vi "Shut_down_EnFlo_Tunnel.vi"(3 "Mode":T5=enum."Run VI", 5 "Traverse line In":T2 {"Carrier_2 Q (l/min)" format="%#.2f"; "Row Duration (mins)" format="%#.1f"; "Row No" min=0; "Trace Gas Concentration (%)" min=0.0 format="%#_4f"; "Carrier_1 Q (l/min)" format="%#.4f"; "Start X" format="%#.2f"; "Start Y" format="%#.2f"; "Start Z" format="%#.2f"; "End X" format="%#.2f"; "End Y" format="%#.2f"; "End Z" format="%#.2f"; "Tunnel Speed" format="%#.2f"; "Averaging time (mins)" min=0.0 format="%#.2f"}) -> (0 "Error Message":string, 1 "Status":T1, 2 "Traverse line Out":T2 {"Carrier_2 Q (l/min)" format="%#.2f"; "Row Duration (mins)" format="%#.1f"; "Row No" min=0; "Trace Gas Concentration (%)" min=0.0 format="%#_4f"; "Carrier_1 Q (l/min)" format="%#.4f"; "Start X" format="%#.2f"; "Start Y" format="%#.2f"; "Start Z" format="%#.2f"; "End X" format="%#.2f"; "End Y" format="%#.2f"; "End Z" format="%#.2f"; "Tunnel Speed" format="%#.2f"; "Averaging time (mins)" min=0.0 format="%#.2f"})   [LabVIEW 2022 SP3]
uses:
  Gen Trav/Traverse_cluster.ctl
  Gen Trav/Spacing.ctl
  Controls/Multi_run_mode.ctl
  Controls/User_Specific_mode.ctl
  Gen Trav/Multi_Run_Status.ctl
  Controls/GMU Gas Line Name.ctl
  ADAM Client/Sub VIs/ADAM Controls/Channel_names.ctl
  ADAM Client/Sub VIs/ADAM Controls/Client_Source_Status.ctl
  ADAM Client/Sub VIs/ADAM Controls/Tunnel_speed_mode.ctl
  Globals/Preference_global.vi
  Globals/Trav_pos_global.vi
panel:
  in  "Stop waiting":bool
  # "X           Y          Z"
  # "Start"
  # "End"
  # "X           Y          Z"
  # "Start"
  # "End"
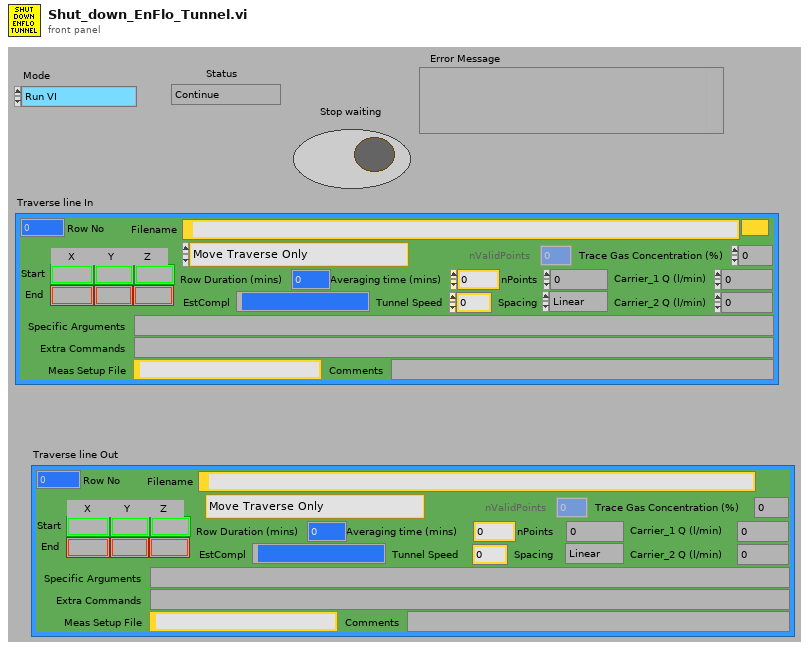
[diagram p1: front panel]
types:
  T1 = typedef "Multi_Run_Status.ctl" = enum16{"Continue", "Continue with Error", "Jump to Next Point", "Jump to Next Row", "Jump To Fall Back", "Terminate Run"}
  T2 = typedef "Traverse_cluster.ctl" = cluster{"Start X":sgl, "Start Y":sgl, "Start Z":sgl, "End X":sgl, "End Y":sgl, "End Z":sgl, "nPoints":i32, "Spacing":T3, "Filename":path, "Tunnel Speed":dbl, "Averaging time (mins)":dbl, "Extra Commands":string, "Carrier_1 Q (l/min)":dbl, "Carrier_2 Q (l/min)":dbl, "Trace Gas Concentration (%)":dbl, "Specific Arguments":string, "Comments":string, "Row No":i32, "Row Type Selector":T4, "EstCompl":string, "Row Duration (mins)":dbl, "nValidPoints":i32, "Meas Setup File":string}
  T3 = typedef "Spacing.ctl" = enum16{"Linear", "Log", "Gauss", "Specified", "N/A"}
  T4 = typedef "Multi_run_mode.ctl" = enum16{"Move Traverse Only", "Set Tunnel Speed Only", "Set Source Only", "Set Measurement Conditions", "Single Measurement", "Vertical Profile", "Lateral Profile", "Longitudinal Profile", "Multi-Axis Profile", "Explore Volume", "Auto Calibrate", "Meas Fast FID Bkgnd", "Check Beam Power", "Scanning Valve Measurement", "Run VI Named:", "Set ADAM Ch", "Wait (minutes)", "Send Message", "Synchronize With:", "Fall Back to this Row", "Turn Off Row Repeating", "Traverse 3D Volume", "Blank Row", "Jump to Fall Back Row"}
  T5 = typedef "User_Specific_mode.ctl" = enum16{"Check VI only", "Run VI"}
  T6 = typedef "GMU Gas Line Name.ctl" = enum16{"GMU1 Source", "GMU2 Source", "GMU2 Calib", "CPP GRC-A", "CPP GRC-B"}
  T7 = typedef "Channel_names.ctl" = enum16{"Active Only", "Active + Off", "All Channels", "Changeable Only", "Always Off", "Always On", "Always Off or On"}
  T8 = typedef "Client_Source_Status.ctl" = enum16{"Not Using", "Using", "Must Have"}
  T9 = typedef "Tunnel_speed_mode.ctl" = enum16{"Set Speed", "Set Speed then wait", "Is tunnel speed allowable?"}
  T10 = cluster{"second":i32, "minute":i32, "hour":i32, "day of month":i32, "month":i32, "year":i32, "day of week":i32, "day of year":i32, "is DST":i32}
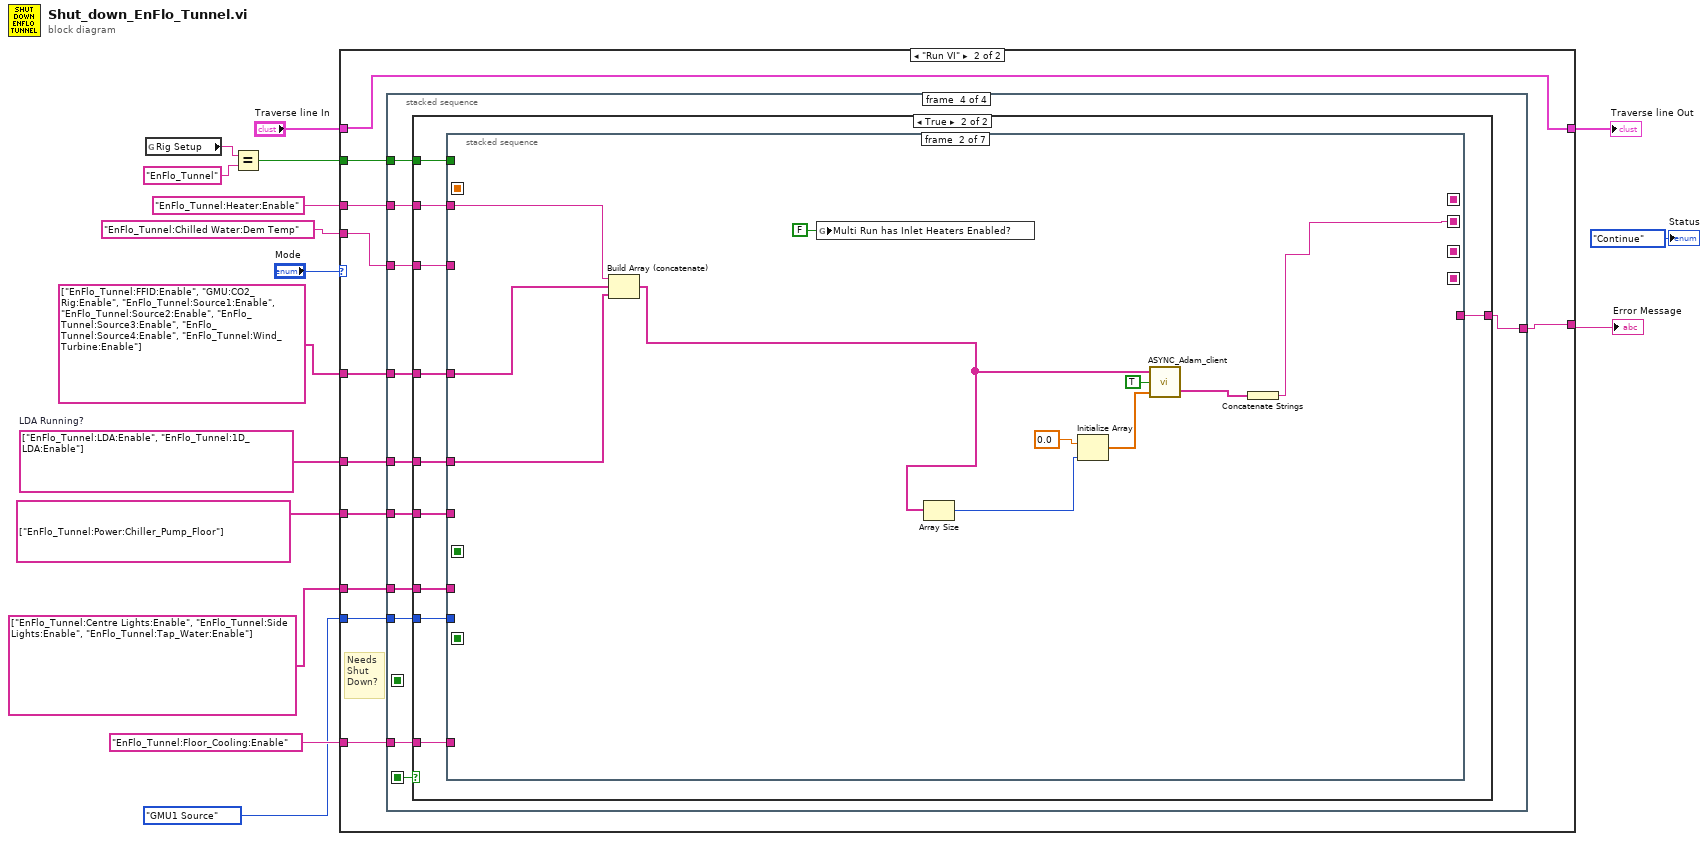
[diagram p0: block diagram]
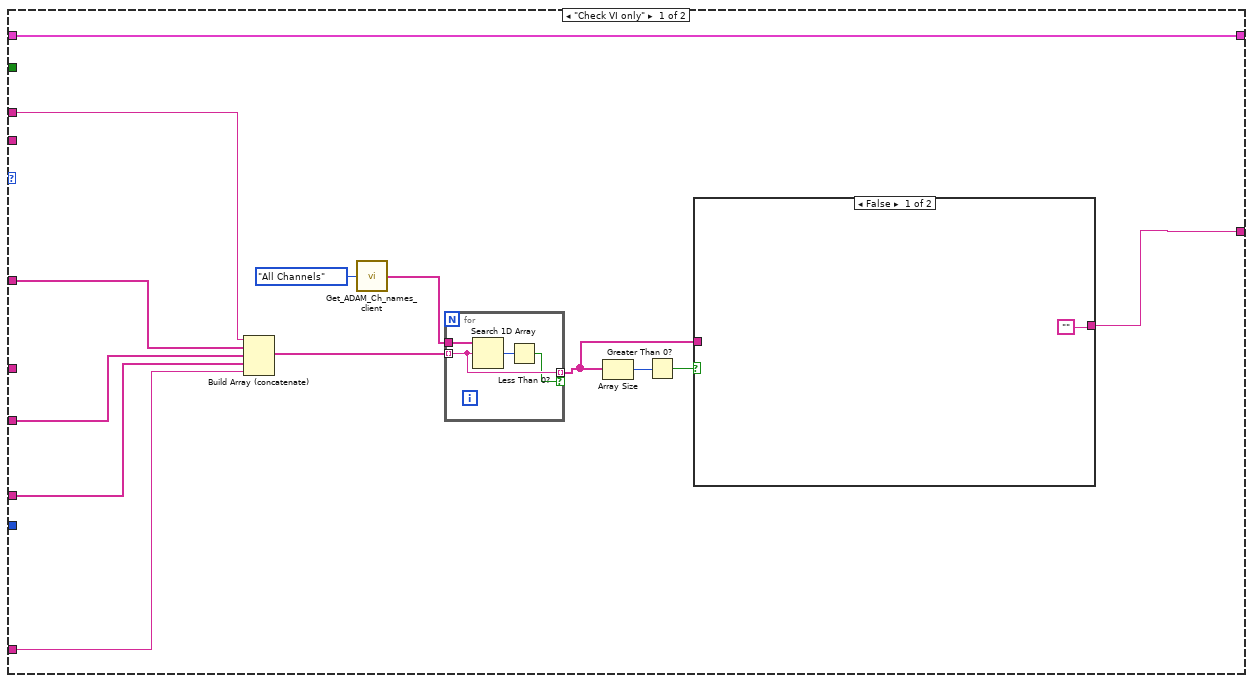
[diagram p2: hidden frame]
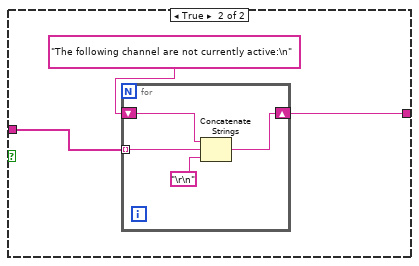
[diagram p3: hidden frame]
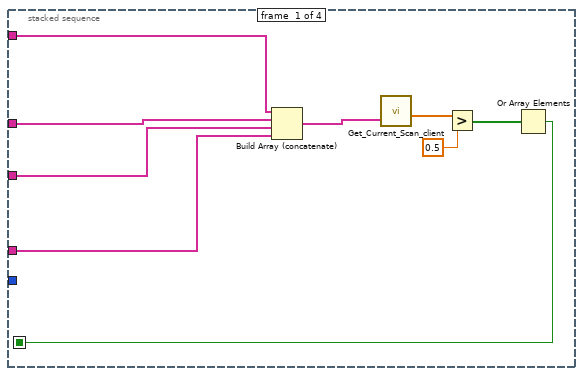
[diagram p4: hidden frame]
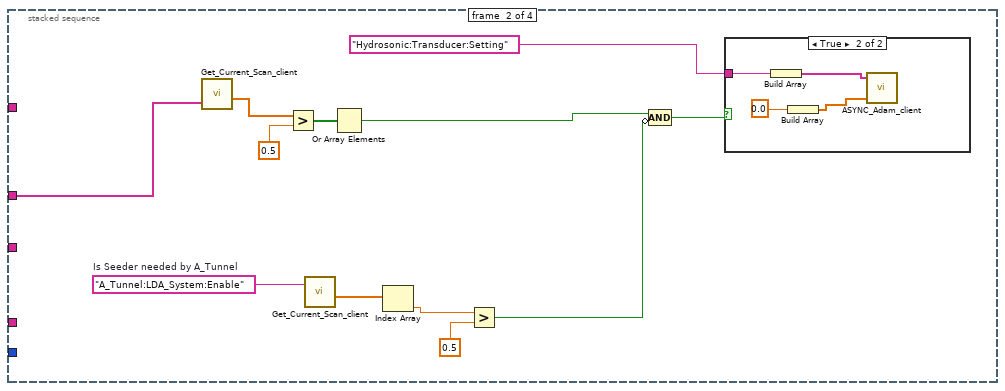
[diagram p5: hidden frame]
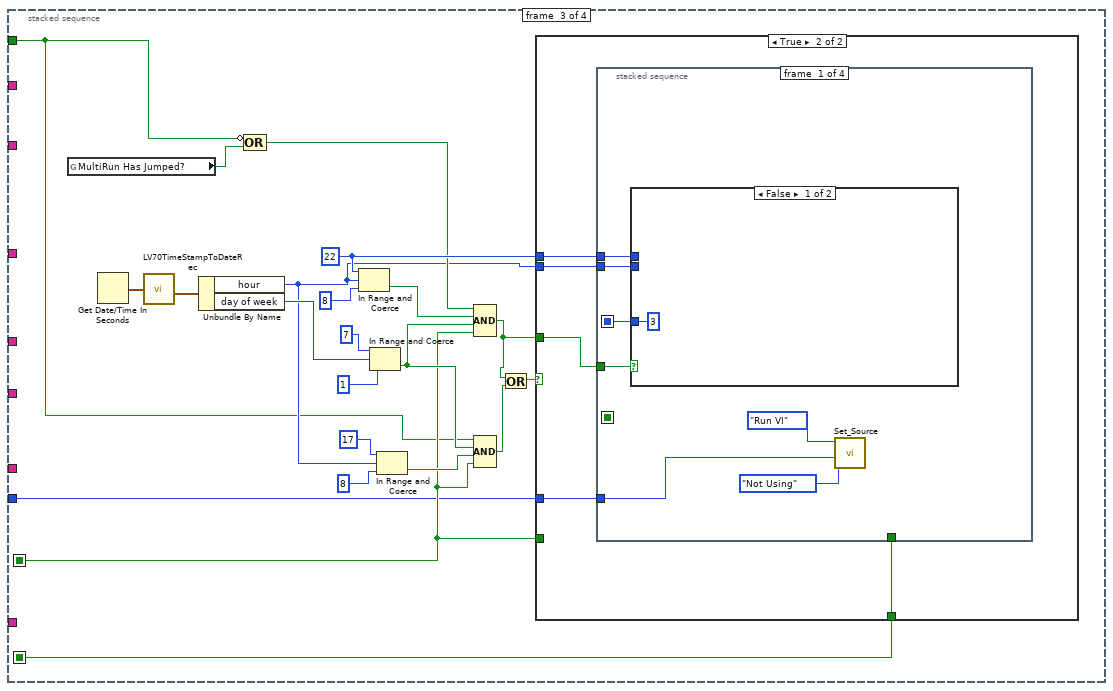
[diagram p7: hidden frame]
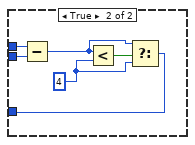
[diagram p9: hidden frame]
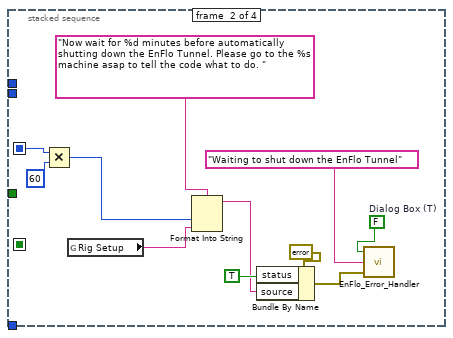
[diagram p10: hidden frame]
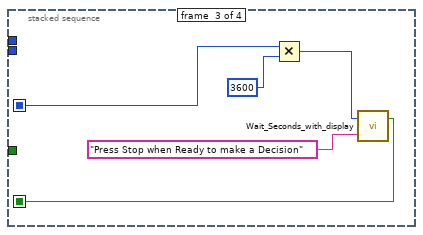
[diagram p11: hidden frame]
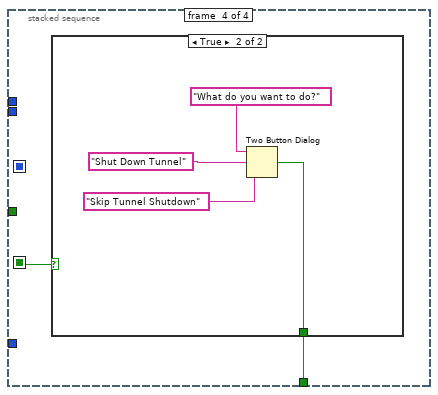
[diagram p12: hidden frame]
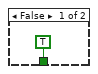
[diagram p13: hidden frame]
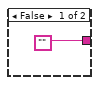
[diagram p14: hidden frame]
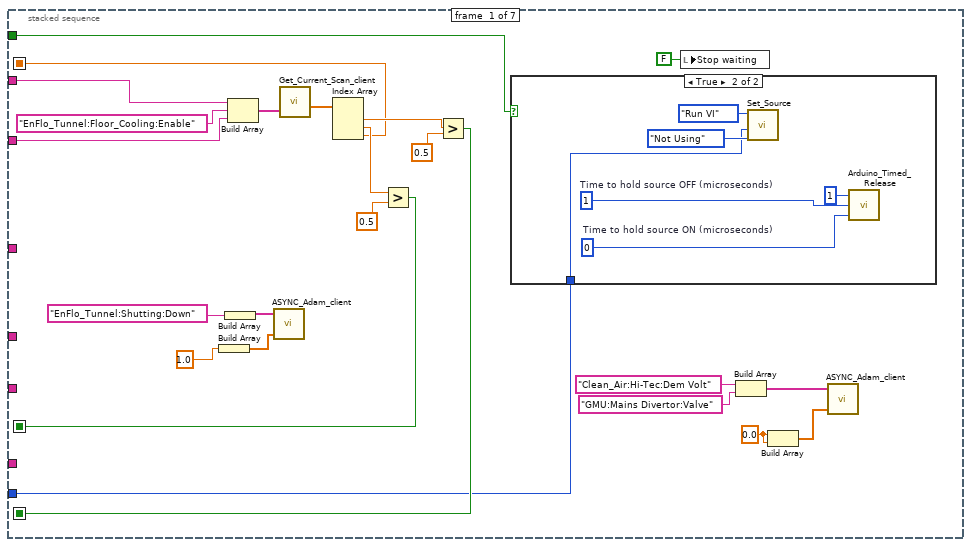
[diagram p15: hidden frame]
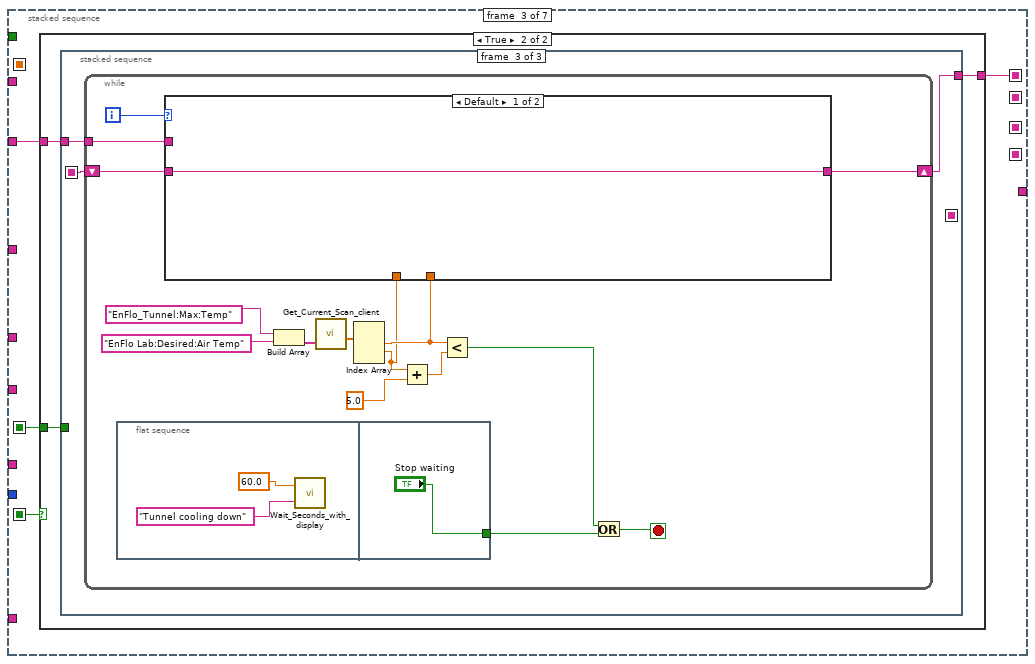
[diagram p17: hidden frame]
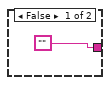
[diagram p18: hidden frame]
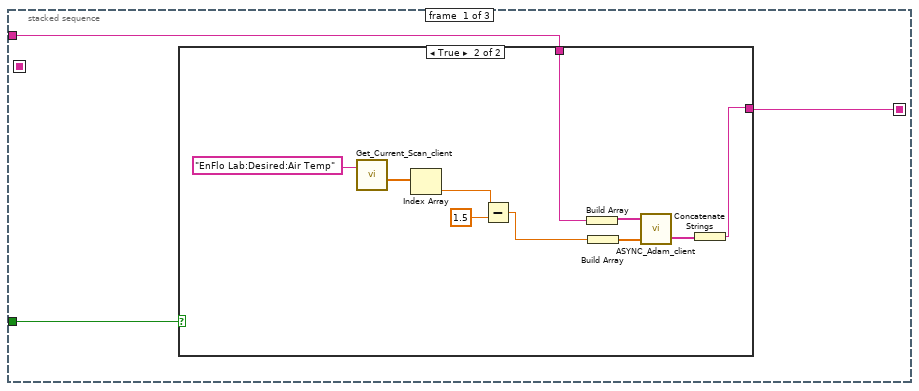
[diagram p19: hidden frame]
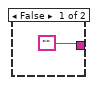
[diagram p20: hidden frame]
diagram:
  w1 = string[] ["EnFlo_Tunnel:LDA:Enable", "EnFlo_Tunnel:1D_LDA:Enable"]  # LDA Running?
  n1 = global read "Preference_global.vi" "Rig Setup"() -> (w5:string)
  n2 = Equal?(x=w5, y="EnFlo_Tunnel" ("Rig Setup")) -> (x = y?=w3:bool)
  n3 = case shown="\"Run VI\"" "Mode" {
    tunnel: "Traverse line In" -> [w29 w52]
    tunnel: [w29 w52] -> w14
    tunnel: [w20 w47] -> w13
    tunnel: "EnFlo_Tunnel:Heater:Enable" -> [w28 w51]
    tunnel: string[] ["EnFlo_Tunnel:FFID:Enable", "GMU:CO2_Rig:Enable", "EnFlo_Tunnel:Source1:Enable", "EnFlo_Tunnel:Source2:Enable", "EnFlo_Tunnel:Source3:Enable", "EnFlo_Tunnel:Source4:Enable", "EnFlo_Tunnel:Wind_Turbine:Enable"] ("appended array") -> [w27 w50]
    tunnel: string[] ["EnFlo_Tunnel:Centre Lights:Enable", "EnFlo_Tunnel:Side Lights:Enable", "EnFlo_Tunnel:Tap_Water:Enable"] ("appended array") -> [w25 w49]
    tunnel: string[] ["EnFlo_Tunnel:Power:Chiller_Pump_Floor"] ("appended array") -> [w26 w48]
    tunnel: "EnFlo_Tunnel:Floor_Cooling:Enable" -> [w17 w46]
    tunnel: "EnFlo_Tunnel:Chilled Water:Dem Temp" -> [_ w45]
    tunnel: w3 -> [_ w44]
    tunnel: GMU_Gas_Line_Name."GMU1 Source" ("Gas Line Name") -> [_ w43]
    tunnel: w1 -> [_ w42]
    frame "Check VI only" {
      n4 = Build Array (concatenate)(w28, w27, w26, w25, w17) -> (w18:string[])
      n5 = call "Get_ADAM_Ch_names_client.vi"("Channel names set"=Channel_names."All Channels") -> ("Ch names"=w19:string[])
      n6 = for {
        tunnel: w19 -> [w41]
        tunnel: w18 -> [w40] mode=indexing
        tunnel: [w40] -> w21 mode=indexing if=w38
        n7 = Search 1D Array(1D array=w41, element=w40) -> (index of element=w39:i32)  [unwired: 1 in]
        n8 = Less Than 0?(x=w39) -> (x < 0?=w38:bool)
      }
      n9 = Array Size(array=w21) -> (size(s)=w23:i32)
      n10 = Greater Than 0?(x=w23) -> (x > 0?=w22:bool)
      n11 = case shown="False" w22 {
        tunnel: w21 -> [_ w33]
        tunnel: ["" w31] -> w20
        frame False {
        }
        frame True {
          n12 = for {
            tunnel: w33 -> [w36] mode=indexing
            shift-right: [w34] -> w31
            shift-left: "The following channel are not currently active:\n" -> [w35]
            n13 = Concatenate Strings(w35, w36, "\r\n") -> (w34:string)
          }
        }
      }
    }
    frame "Run VI" {
      # "Needs\nShut\nDown?"
      n14 = stacked-sequence {
        seq-local: [_ _ w91 _] -> [_ _ _ w148]
        seq-local: [w54 _ _ _] -> [_ _ w83 _]
        tunnel: w51 -> [_ _ _ w153]
        tunnel: w50 -> [w61 _ _ w152]
        tunnel: w49 -> [w59 _ _ w151]
        tunnel: w48 -> [w60 _ _ w150]
        tunnel: [_ _ _ w149] -> w47
        tunnel: w46 -> [_ _ _ w147]
        tunnel: w45 -> [_ _ _ w146]
        tunnel: w44 -> [_ _ w82 w145]
        tunnel: w43 -> [_ _ w78 w144]
        tunnel: w42 -> [w53 w70 _ w143]
        frame #0 {
          n15 = Build Array (concatenate)(w61, w53, w60, w59) -> (w58:string[])
          n16 = call "Get_Current_Scan_client.vi"("multipleChannels"=w58) -> ("Numerical Values"=w57:dbl[])  [unwired: 1 in, 3 out]
          n17 = Greater?(x=w57, y=0.5) -> (0:w55:bool[])
          n18 = Or Array Elements(Boolean array=w55) -> (logical OR=w54:bool)
        }
        frame #1 {
          w68 = "A_Tunnel:LDA_System:Enable"  # Is Seeder needed by A_Tunnel
          n19 = call "Get_Current_Scan_client.vi"("multipleChannels"=w70) -> ("Numerical Values"=w72:dbl[])  [unwired: 1 in, 3 out]
          n20 = Greater?(x=w72, y=0.5) -> (0:w69:bool[])
          n21 = call "Get_Current_Scan_client.vi"("singleChannel"=w68) -> ("Numerical Values"=w66:dbl[])  [unwired: 1 in, 3 out]
          n22 = Or Array Elements(Boolean array=w69) -> (logical OR=w67:bool)
          n23 = Index Array(array=w66) -> (element=w64:dbl)  [unwired: 1 in]
          n24 = Greater?(x=w64, y=0.5) -> (0:w63:bool)
          n25 = Compound Arithmetic op=AND(w67, invert w63) -> (w73:bool)
          n26 = case shown="True" w73 {
            tunnel: "Hydrosonic:Transducer:Setting" -> [_ w77]
            frame False {
            }
            frame True {
              n27 = Build Array(w77) -> (w76:string[])
              n28 = Build Array(0.0) -> (w75:dbl[])
              n29 = call "ASYNC_Adam_client.vi"("Values"=w75, "Channel Names"=w76) -> ()  [unwired: 1 in, 2 out]
            }
          }
        }
        frame #2 {
          w92 = 22 ("lower limit")
          n30 = global read "Trav_pos_global.vi" "MultiRun Has Jumped?"() -> (w90:bool)
          n31 = Get Date/Time In Seconds() -> (seconds since 1Jan1904=w96:timestamp)
          n32 = call <vilib>:"LV70TimeStampToDateRec.vi"("time stamp"=w96) -> ("date time rec"=w99:T10)
          n33 = Unbundle By Name(w99) -> ("hour"=w85:i32, "day of week"=w95:i32)
          n34 = Compound Arithmetic op=OR(invert w82, w90) -> (w89:bool)
          n35 = In Range and Coerce(upper limit=w92, x=w85, lower limit=8) -> (In Range?=w93:bool)  [unwired: 1 out]
          n36 = In Range and Coerce(upper limit=7, x=w95, lower limit=1) -> (In Range?=w88:bool)  [unwired: 1 out]
          n37 = In Range and Coerce(upper limit=17 ("lower limit"), x=w85, lower limit=8) -> (In Range?=w84:bool)  [unwired: 1 out]
          n38 = Compound Arithmetic op=AND(w89, w93, w88, w83) -> (w79:bool)
          n39 = Compound Arithmetic op=AND(w82, w88, w84, w83) -> (w80:bool)
          n40 = Or(x=w79, y=w80) -> (x .or. y?=w81:bool)
          n41 = case shown="True" w81 {
            tunnel: w92 -> [_ w105]
            tunnel: w85 -> [_ w104]
            tunnel: [w100 w103] -> w91
            tunnel: w83 -> [w100 _]
            tunnel: w79 -> [_ w102]
            tunnel: w78 -> [_ w101]
            frame False {
            }
            frame True {
              n42 = stacked-sequence {
                seq-local: [_ _ w132 _] -> [_ _ _ w136]
                seq-local: [w110 _ _ _] -> [_ w125 w131 _]
                tunnel: w105 -> [w112 _ _ _]
                tunnel: w104 -> [w111 _ _ _]
                tunnel: [_ _ _ w137] -> w103
                tunnel: w102 -> [w107 _ _ _]
                tunnel: w101 -> [w106 _ _ _]
                frame #0 {
                  n43 = case shown="False" w107 {
                    tunnel: w112 -> [_ w119]
                    tunnel: w111 -> [_ w118]
                    tunnel: [3 ("y") w114] -> w110
                    frame False {
                    }
                    frame True {
                      w115 = 4 ("y")
                      n44 = Subtract(x=w119, y=w118) -> (x-y=w116:i32)
                      n45 = Less?(x=w116, y=w115) -> (x < y?=w117:bool)
                      n46 = Select(t=w116, s=w117, f=w115) -> (s? t:f=w114:i32)
                    }
                  }
                  n47 = call "Set_Source.vi"("Source Status"=Client_Source_Status."Not Using", "Gas Line Name"=w106, "Simulate/Run"=User_Specific_mode."Run VI") -> ()  [unwired: 2 in, 6 out]
                }
                frame #1 {
                  w128 = FALSE  # Dialog Box (T)
                  n48 = Multiply(x=w125, y=60) -> (x*y=w122:i32)
                  n49 = global read "Preference_global.vi" "Rig Setup"() -> (w121:string)
                  n50 = Format Into String(format string="Now wait for %d minutes before automatically shutting down the EnFlo Tunnel. Please go to the %s machine asap to tell the code what to do. ", w122, w121) -> (resulting string=w120:string)  [unwired: 2 in, 1 out]
                  n51 = Bundle By Name(cluster=errorcluster {"status"=FALSE, "code"=0, "source"=""} ("error in (no error)"), "status"=TRUE ("Bundle Element"), "source"=w120) -> (w130:errorcluster)
                  n52 = call "EnFlo_Error_Handler.vi"("error in (no error)"=w130, "Error Type"="Waiting to shut down the EnFlo Tunnel", "Dialog Box (F)"=w128) -> ()  [unwired: 3 out]
                }
                frame #2 {
                  n53 = Multiply(x=w131, y=3600) -> (x*y=w133:i32)
                  n54 = call "Wait_Seconds_with_display.vi"("Message"="Press Stop when Ready to make a Decision", "Seconds to wait"=w133) -> ("Stopped"=w132:bool)  [unwired: 1 out]
                }
                frame #3 {
                  n55 = case shown="True" w136 {
                    tunnel: [TRUE ("T button?") w139] -> w137
                    frame False {
                    }
                    frame True {
                      n56 = Two Button Dialog(message="What do you want to do?", 1:"Skip Tunnel Shutdown" ("F button name (\"Cancel\")"), 2:"Shut Down Tunnel" ("T button name (\"OK\")")) -> (T button?=w139:bool)
                    }
                  }
                }
              }
            }
          }
        }
        frame #3 {
          n57 = case shown="True" w148 {
            tunnel: w153 -> [_ w164]
            tunnel: w152 -> [_ w163]
            tunnel: w151 -> [_ w162]
            tunnel: w150 -> [_ w161]
            tunnel: ["" w160] -> w149
            tunnel: w147 -> [_ w159]
            tunnel: w146 -> [_ w158]
            tunnel: w145 -> [_ w157]
            tunnel: w144 -> [_ w156]
            tunnel: w143 -> [_ w155]
            frame False {
            }
            frame True {
              n58 = stacked-sequence {
                seq-local: [w184 _ _ _ _ _ _] -> [_ _ w209 _ _ _ _]
                seq-local: [_ w201 _ _ _ _ _] -> [_ _ _ _ w292 _ _]
                seq-local: [_ _ _ w271 _ _ _] -> [_ _ _ _ w293 _ _]
                seq-local: [_ _ _ w269 _ _ _] -> [_ _ _ _ w289 _ _]
                seq-local: [w178 _ _ _ _ _ _] -> [_ _ w208 _ _ _ _]
                seq-local: [w172 _ _ _ _ _ _] -> [_ _ _ _ _ _ w318]
                seq-local: [_ _ w206 _ _ _ _] -> [_ _ _ _ w284 _ _]
                tunnel: w164 -> [w183 w200 _ _ _ _ _]
                tunnel: w163 -> [_ w199 _ _ _ w309 _]
                tunnel: w162 -> [_ _ _ _ w287 w307 _]
                tunnel: w161 -> [_ _ _ w273 _ w308 _]
                tunnel: [_ _ _ _ w291 _ _] -> w160
                tunnel: w159 -> [_ _ _ _ w288 _ _]
                tunnel: w158 -> [w173 _ w207 _ _ _ w319]
                tunnel: w157 -> [w166 _ _ _ _ _ _]
                tunnel: w156 -> [w165 _ _ _ _ _ _]
                tunnel: w155 -> [_ w196 _ _ _ w297 _]
                frame #0 {
                  w168 = 0.0 ("element")
                  n59 = Build Array(1.0) -> (w175:dbl[])
                  n60 = Build Array("EnFlo_Tunnel:Shutting:Down") -> (w176:string[])
                  n61 = Build Array(w183, "EnFlo_Tunnel:Floor_Cooling:Enable", w173) -> (w188:string[])
                  n62 = call "ASYNC_Adam_client.vi"("Values"=w175, "Channel Names"=w176) -> ()  [unwired: 1 in, 2 out]
                  n63 = call "Get_Current_Scan_client.vi"("multipleChannels"=w188) -> ("Numerical Values"=w187:dbl[])  [unwired: 1 in, 3 out]
                  n64 = Index Array(array=w187) -> (element #1=w186:dbl, element #2=w179:dbl, element #3=w172:dbl)  [unwired: 3 in]
                  n65 = Greater?(x=w179, y=0.5) -> (0:w178:bool)
                  n66 = Greater?(x=w186, y=0.5) -> (0:w184:bool)
                  n67 = case shown="True" w166 {
                    tunnel: w165 -> [_ w189]
                    frame False {
                    }
                    frame True {
                      w193 = u32 1  # Time to hold source OFF (microseconds)
                      w192 = u32 0  # Time to hold source ON (microseconds)
                      n68 = call "Set_Source.vi"("Source Status"=Client_Source_Status."Not Using", "Gas Line Name"=w189, "Simulate/Run"=User_Specific_mode."Run VI") -> ()  [unwired: 2 in, 6 out]
                      n69 = call "Arduino_Timed_Release.vi"("Time to hold source ON (microseconds)"=w192, "Time to hold source OFF (microseconds)"=w193, "Number of cycles"=u16 1) -> ()  [unwired: 2 out]
                    }
                  }
                  n70 = local write "Stop waiting"(FALSE ("Stop waiting")) -> ()
                  n71 = Build Array("Clean_Air:Hi-Tec:Dem Volt", "GMU:Mains Divertor:Valve") -> (w170:string[])
                  n72 = Build Array(w168, w168) -> (w169:dbl[])
                  n73 = call "ASYNC_Adam_client.vi"("Values"=w169, "Channel Names"=w170) -> ()  [unwired: 1 in, 2 out]
                }
                frame #1 {
                  n74 = Build Array (concatenate)(w200, w199, w196) -> (w198:string[])
                  n75 = global write "Trav_pos_global.vi" "Multi Run has Inlet Heaters Enabled?"(FALSE ("Multi Run has Inlet Heaters Enabled?")) -> ()
                  n76 = Array Size(array=w198) -> (size(s)=w205:i32)
                  n77 = Initialize Array(0.0 ("Input Element"), w205) -> (w204:dbl[])
                  n78 = call "ASYNC_Adam_client.vi"("Values"=w204, "Check Value is in the scan table?"=TRUE, "Channel Names"=w198) -> ("Scan Comments"=w202:string[])  [unwired: 1 out]
                  n79 = Concatenate Strings(w202) -> (w201:string)
                }
                frame #2 {
                  n80 = case shown="True" w209 {
                    tunnel: w208 -> [_ w213]
                    tunnel: w207 -> [_ w212]
                    tunnel: ["" w211] -> w206
                    frame False {
                    }
                    frame True {
                      n81 = stacked-sequence {
                        seq-local: [w214 _ _] -> [_ w229 _]
                        seq-local: [_ w228 _] -> [_ _ w233]
                        tunnel: w213 -> [w216 _ _]
                        tunnel: w212 -> [w215 _ w234]
                        tunnel: [_ _ w232] -> w211
                        frame #0 {
                          n82 = case shown="True" w216 {
                            tunnel: w215 -> [_ w221]
                            tunnel: ["" w218] -> w214
                            frame False {
                            }
                            frame True {
                              n83 = call "Get_Current_Scan_client.vi"("singleChannel"="EnFlo Lab:Desired:Air Temp") -> ("Numerical Values"=w226:dbl[])  [unwired: 1 in, 3 out]
                              n84 = Index Array(array=w226) -> (element=w222:dbl)  [unwired: 1 in]
                              n85 = Subtract(x=w222, y=1.5) -> (x-y=w224:dbl)
                              n86 = Build Array(w221) -> (w225:string[])
                              n87 = Build Array(w224) -> (w223:dbl[])
                              n88 = call "ASYNC_Adam_client.vi"("Values"=w223, "Channel Names"=w225) -> ("Scan Comments"=w219:string[])  [unwired: 1 in, 1 out]
                              n89 = Concatenate Strings(w219) -> (w218:string)
                            }
                          }
                        }
                        frame #1 {
                          n90 = call "Set EnFlo Tunnel inlet Fans.vi"("Tunnel Velocity m/s"=0.0) -> ("Error Message"=w230:string)
                          n91 = Concatenate Strings(w229, w230) -> (w228:string)
                        }
                        frame #2 {
                          n92 = while {
                            tunnel: w234 -> [w237]
                            shift-right: [w235] -> w232
                            shift-left: w233 -> [w236]
                            i -> [w240]
                            stop <- w242 stop-if-true
                            n93 = flat-sequence {
                              tunnel: ["Stop waiting"] -> w241
                              frame #0 {
                                n94 = call "Wait_Seconds_with_display.vi"("Message"="Tunnel cooling down", "Seconds to wait"=60.0) -> ()  [unwired: 2 out]
                              }
                              frame #1 {
                              }
                            }
                            n95 = Build Array("EnFlo_Tunnel:Max:Temp", "EnFlo Lab:Desired:Air Temp") -> (w247:string[])
                            n96 = call "Get_Current_Scan_client.vi"("multipleChannels"=w247) -> ("Numerical Values"=w248:dbl[])  [unwired: 1 in, 3 out]
                            n97 = Index Array(array=w248) -> (element #1=w239:dbl, element #2=w238:dbl)  [unwired: 3 in, 1 out]
                            n98 = case shown="Default" w240 {
                              tunnel: w239 -> [_ w260]
                              tunnel: w238 -> [_ w255]
                              tunnel: w237 -> [_ w254]
                              tunnel: w236 -> [w250 w252]
                              tunnel: [w250 w251] -> w235
                              frame Default {
                              }
                              frame 30 {
                                w265 = FALSE  # Dialog Box (T)
                                n99 = Build Array(w254) -> (w257:string[])
                                n100 = Build Array(w255) -> (w256:dbl[])
                                n101 = call "ASYNC_Adam_client.vi"("Values"=w256, "Channel Names"=w257) -> ("Scan Comments"=w253:string[])  [unwired: 1 in, 1 out]
                                n102 = Concatenate Strings(w252, w253) -> (w251:string)
                                n103 = Format Into String(format string="EnFlo_Tunnel:Max:Temp is now %.1f.", w260) -> (resulting string=w258:string)  [unwired: 2 in, 1 out]
                                n104 = Bundle By Name(cluster=errorcluster {"status"=FALSE, "code"=0, "source"=""} ("error in (no error)"), "status"=TRUE ("Bundle Element"), "source"=w258) -> (w264:errorcluster)
                                n105 = call "EnFlo_Error_Handler.vi"("error in (no error)"=w264, "Error Type"="Waiting for the EnFlo Tunnel to cool down", "Dialog Box (F)"=w265) -> ()  [unwired: 3 out]
                              }
                            }
                            n106 = Add(x=w238, y=5.0) -> (x+y=w244:dbl)
                            n107 = Less?(x=w239, y=w244) -> (x < y?=w243:bool)
                            n108 = Or(x=w243, y=w241) -> (x .or. y?=w242:bool)
                          }
                        }
                      }
                    }
                  }
                }
                frame #3 {
                  n109 = Array Size(array=w273) -> (size(s)=w276:i32)
                  n110 = for {
                    N: 10 -> [_]
                    tunnel: [w278] -> w269
                    stop <- w279 stop-if-true
                    n111 = call "Set_Tunnel_Speed.vi"("Mode"=Tunnel_speed_mode."Set Speed then wait", "Rig Name (default Empty)"="EnFlo_Tunnel", "Tunnel Velocity m/s"=0.0) -> ("Error String"=w278:string)  [unwired: 1 in, 1 out]
                    n112 = Empty String/Path?(string/path=w278) -> (empty?=w279:bool)
                    n113 = case shown="False" w279 {
                      tunnel: w278 -> [w282 _]
                      frame False {
                        n114 = call "Wait_Seconds_with_display.vi"("Message"=w282, "Seconds to wait"=60.0) -> ()  [unwired: 2 out]
                      }
                      frame True {
                      }
                    }
                  }
                  n115 = Initialize Array(0.0 ("Input Element"), w276) -> (w274:dbl[])
                  n116 = call "ASYNC_Adam_client.vi"("Values"=w274, "Channel Names"=w273) -> ("Scan Comments"=w272:string[])  [unwired: 1 in, 1 out]
                  n117 = Concatenate Strings(w272) -> (w271:string)
                }
                frame #4 {
                  n118 = Build Array (concatenate)(w287, w288) -> (w286:string[])
                  n119 = Array Size(array=w286) -> (size(s)=w296:i32)
                  n120 = Initialize Array(0.0 ("Input Element"), w296) -> (w295:dbl[])
                  n121 = call "ASYNC_Adam_client.vi"("Values"=w295, "Check Value is in the scan table?"=TRUE, "Channel Names"=w286) -> ("Scan Comments"=w285:string[])  [unwired: 1 out]
                  n122 = Concatenate Strings(w289, w293, w292, w284, w285) -> (w291:string)
                }
                frame #5 {
                  w302 = FALSE  # Dialog Box (T)
                  n123 = Build Array (concatenate)(string[] ["EnFlo_Tunnel:Reference:Velocity"] ("appended array"), w309, w297, w308, w307) -> (w306:string[])
                  n124 = call "Get_Current_Scan_client.vi"("multipleChannels"=w306) -> ("Numerical Values"=w303:dbl[])  [unwired: 1 in, 3 out]
                  n125 = for {
                    tunnel: w306 -> [w317] mode=indexing
                    shift-right: [w314] -> w304
                    shift-left: "\nStatus Report\n" -> [w315]
                    tunnel: w303 -> [w313] mode=indexing
                    n126 = call "Number_2_string.vi"("precision"="2", "number"=w313) -> ("String"=w311:string)
                    n127 = Format Into String(format string="%s   =  %s\n", initial string=w315, w317, w311) -> (resulting string=w314:string)  [unwired: 1 in, 1 out]
                  }
                  n128 = Bundle By Name(cluster=errorcluster {"status"=FALSE, "code"=0, "source"=""} ("error in (no error)"), "status"=TRUE ("Bundle Element"), "source"=w304) -> (w301:errorcluster)
                  n129 = call "EnFlo_Error_Handler.vi"("error in (no error)"=w301, "Error Type"="Successful Shut Down of the EnFlo Tunnel", "Dialog Box (F)"=w302) -> ()  [unwired: 3 out]
                }
                frame #6 {
                  n130 = Build Array(w319) -> (w321:string[])
                  n131 = Build Array(w318) -> (w320:dbl[])
                  n132 = call "ASYNC_Adam_client.vi"("Values"=w320, "Channel Names"=w321) -> ()  [unwired: 1 in, 2 out]
                }
              }
            }
          }
        }
      }
    }
  }
  "Traverse line Out" <- w14
  "Error Message" <- w13
  "Status" <- Multi_Run_Status."Continue" ("Status")
